vi "mapSubDataSVToUE.vi"(6 "Time Stamp":timestamp, 8 "error in (no error)":errorcluster, 9 "svValue":variant, 10 "svArrayIndex":i32, 11 "MiddlewareSVThisComponent in":refnum<class "MiddlewareSVThisComponent.lvclass">) -> (0 "error out":errorcluster, 3 "MiddlewareSVThisComponent out":refnum<class "MiddlewareSVThisComponent.lvclass">)   [LabVIEW 2015, in "MiddlewareSVThisComponent.lvclass"]
uses:
  MiddlewareSVThisComponent.lvclass
  MiddlewareSVThisComponent.lvclass/MiddlewareSVThisComponent.ctl
  PubSubDataEvent/PubSubDataEvent.lvclass/PubSubDataEvent.ctl
  PubSubDataEvent/PubSubDataEvent.lvclass
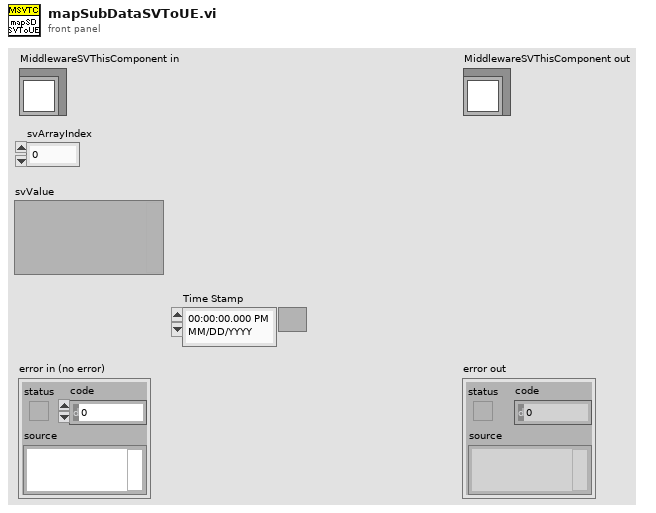
[diagram p1: front panel]
types:
  T1 = typedef "EXATypedefs.lvlib/SubDataSV.ctl" = enum16{"ClearError", "Disable", "Enable", "Exit", "GoToStandby", "HeartbeatIn", "Start"}
  T2 = typedef "EXATypedefs.lvlib/SubDataEvents.ctl" = cluster{"ClearError":refnum<user-event>, "Disable":refnum<user-event>, "Enable":refnum<user-event>, "Exit":refnum<user-event>, "GoToStandby":refnum<user-event>, "HeartbeatIn":refnum<user-event>, "Start":refnum<user-event>}
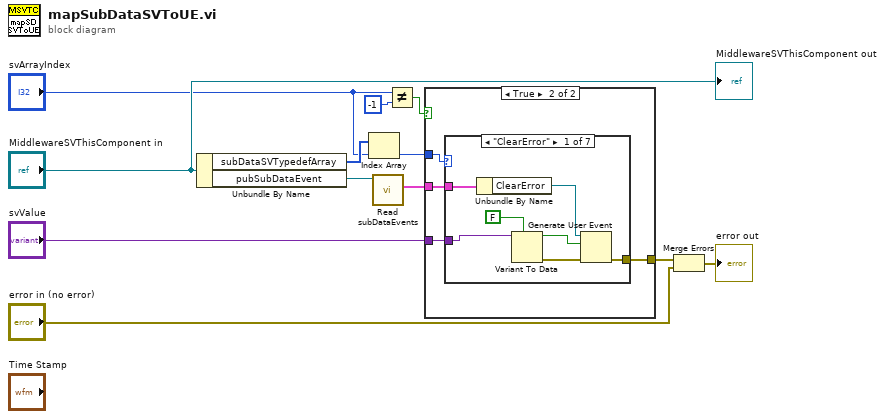
[diagram p0: block diagram]
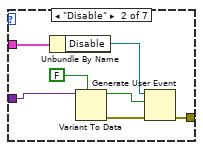
[diagram p3: hidden frame]
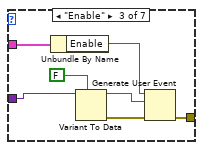
[diagram p4: hidden frame]
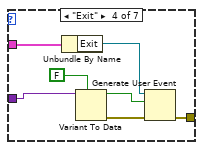
[diagram p5: hidden frame]
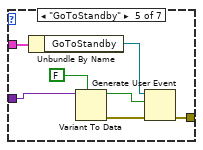
[diagram p6: hidden frame]
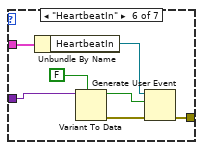
[diagram p7: hidden frame]
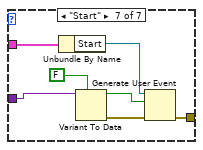
[diagram p8: hidden frame]
diagram:
  n1 = Unbundle By Name("MiddlewareSVThisComponent in") -> ("subDataSVTypedefArray"=w12:T1[], "pubSubDataEvent"=w8:refnum<class "PubSubDataEvent.lvclass">)
  n2 = Index Array(array=w12, index="svArrayIndex") -> (element=w11:T1)
  n3 = call "Read subDataEvents.vi"("PubSubDataEvent in"=w8) -> ("SubDataEvents"=w7:T2)  [unwired: 9 in, 1 out]
  n4 = Not Equal?(x="svArrayIndex", y=-1) -> (x != y?=w9:bool)
  n5 = case shown="True" w9 {
    tunnel: "svValue" -> [_ w14]
    tunnel: w11 -> [_ w16]
    tunnel: w7 -> [_ w15]
    tunnel: [_ w13] -> w1
    frame False {
    }
    frame True {
      n6 = case shown="\"ClearError\"" w16 {
        tunnel: w14 -> [w21 w28 w35 w42 w49 w56 w63]
        tunnel: w15 -> [w23 w30 w37 w44 w51 w58 w65]
        tunnel: [w17 w24 w31 w38 w45 w52 w59] -> w13
        frame "ClearError" {
          n7 = Unbundle By Name(w23) -> ("ClearError"=w22:refnum<user-event>)
          n8 = Variant To Data(type=FALSE ("event data"), Variant=w21) -> (data=w19:bool, error out=w18:errorcluster)  [unwired: 1 in]
          n9 = Generate User Event(user event=w22, event data cluster=w19, error in=w18) -> (error out=w17:errorcluster)  [unwired: 1 in, 1 out]
        }
        frame "Disable" {
          n10 = Unbundle By Name(w30) -> ("Disable"=w29:refnum<user-event>)
          n11 = Variant To Data(type=FALSE ("event data"), Variant=w28) -> (data=w26:bool, error out=w25:errorcluster)  [unwired: 1 in]
          n12 = Generate User Event(user event=w29, event data cluster=w26, error in=w25) -> (error out=w24:errorcluster)  [unwired: 1 in, 1 out]
        }
        frame "Enable" {
          n13 = Unbundle By Name(w37) -> ("Enable"=w36:refnum<user-event>)
          n14 = Variant To Data(type=FALSE ("event data"), Variant=w35) -> (data=w33:bool, error out=w32:errorcluster)  [unwired: 1 in]
          n15 = Generate User Event(user event=w36, event data cluster=w33, error in=w32) -> (error out=w31:errorcluster)  [unwired: 1 in, 1 out]
        }
        frame "Exit" {
          n16 = Unbundle By Name(w44) -> ("Exit"=w43:refnum<user-event>)
          n17 = Variant To Data(type=FALSE ("event data"), Variant=w42) -> (data=w40:bool, error out=w39:errorcluster)  [unwired: 1 in]
          n18 = Generate User Event(user event=w43, event data cluster=w40, error in=w39) -> (error out=w38:errorcluster)  [unwired: 1 in, 1 out]
        }
        frame "GoToStandby" {
          n19 = Unbundle By Name(w51) -> ("GoToStandby"=w50:refnum<user-event>)
          n20 = Variant To Data(type=FALSE ("event data"), Variant=w49) -> (data=w47:bool, error out=w46:errorcluster)  [unwired: 1 in]
          n21 = Generate User Event(user event=w50, event data cluster=w47, error in=w46) -> (error out=w45:errorcluster)  [unwired: 1 in, 1 out]
        }
        frame "HeartbeatIn" {
          n22 = Unbundle By Name(w58) -> ("HeartbeatIn"=w57:refnum<user-event>)
          n23 = Variant To Data(type=FALSE ("event data"), Variant=w56) -> (data=w54:bool, error out=w53:errorcluster)  [unwired: 1 in]
          n24 = Generate User Event(user event=w57, event data cluster=w54, error in=w53) -> (error out=w52:errorcluster)  [unwired: 1 in, 1 out]
        }
        frame "Start" {
          n25 = Unbundle By Name(w65) -> ("Start"=w64:refnum<user-event>)
          n26 = Variant To Data(type=FALSE ("event data"), Variant=w63) -> (data=w61:bool, error out=w60:errorcluster)  [unwired: 1 in]
          n27 = Generate User Event(user event=w64, event data cluster=w61, error in=w60) -> (error out=w59:errorcluster)  [unwired: 1 in, 1 out]
        }
      }
    }
  }
  n28 = Merge Errors(w1, "error in (no error)") -> (→"error out":errorcluster)
  "MiddlewareSVThisComponent out" <- "MiddlewareSVThisComponent in"
